vi "Actor Core.vi"(8 "error in":errorcluster, 11 "Interactive Tree in":refnum<class "Interactive Tree.lvclass">) -> (0 "error out":errorcluster, 3 "Actor out":refnum<class "Actor.lvclass">)   [LabVIEW 2016, in "Interactive Tree.lvclass"]
doc: "(<B>Filename</B>: Actor Framework.lvlib:Actor.lvclass:Actor Core.vi)\n\nReceives messages to the actor, reacts to them, and initiates any error handling that may shut the actor down.\n\nDescendant classes may override this VI to append parallel tasks for the actor to complete while it handles messages. Overrides use the Call Parent Method node."
uses:
  Interactive Tree.lvclass
  D:/github/Measure_core/Measure Object/Measure Object.lvclass
  D:/Program Files/National Instruments/LabVIEW 2016/vi.lib/ActorFramework/Actor/Actor.lvclass
  <vilib>/ActorFramework/Actor/Actor.lvclass
  Interactive Tree.lvclass/Interactive Tree.ctl
  Measure Object/Measure Object.lvclass/Measure Object.ctl
  <vilib>/ActorFramework/Actor/Actor.lvclass/Actor.ctl
  <vilib>/ActorFramework/Message Enqueuer/Message Enqueuer.lvclass/Message Enqueuer.ctl
  Interactive Tree Messages/Insert Item Msg/Insert Item Msg.lvclass/Insert Item Msg.ctl
  Measure Object/Read stop event.vi
  <vilib>/ActorFramework/Message Enqueuer/Init from Existing Queue.vi
  <vilib>/ActorFramework/Message Enqueuer/Enqueue.vi
  Interactive Tree Messages/Insert Item Msg/Insert Item Msg.lvclass
  D:/Program Files/National Instruments/LabVIEW 2016/vi.lib/ActorFramework/Message/Message.lvclass
  <vilib>/ActorFramework/Message Priority Queue/Priority Enqueue.vi
  <vilib>/ActorFramework/Message Enqueuer/Message Enqueuer.lvclass
  Measure Object/Measure Object.lvclass
panel:
  in  "Items":i32(listbox)
  in  "Tree":string(tree)
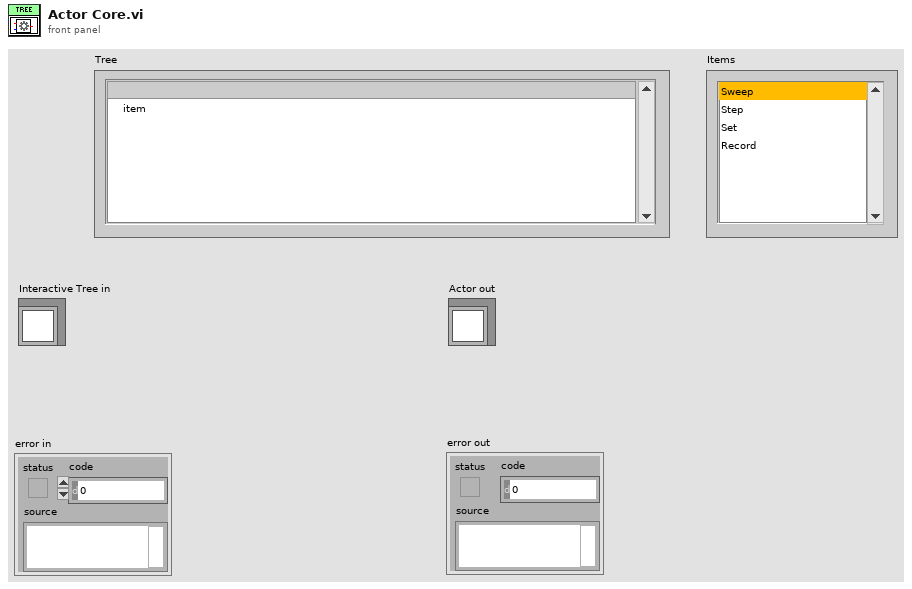
[diagram p1: front panel]
types:
  T1 = typedef "imagedata.ctl" = cluster{"image type":i32, "image depth":i32, "image":u8[], "mask":u8[], "colors":u32[], "Rectangle":cluster{"left":i16, "top":i16, "right":i16, "bottom":i16}}
  T2 = typedef "LVPoint32TypeDef.ctl" = cluster{"Horizontal":i32, "Vertical":i32}
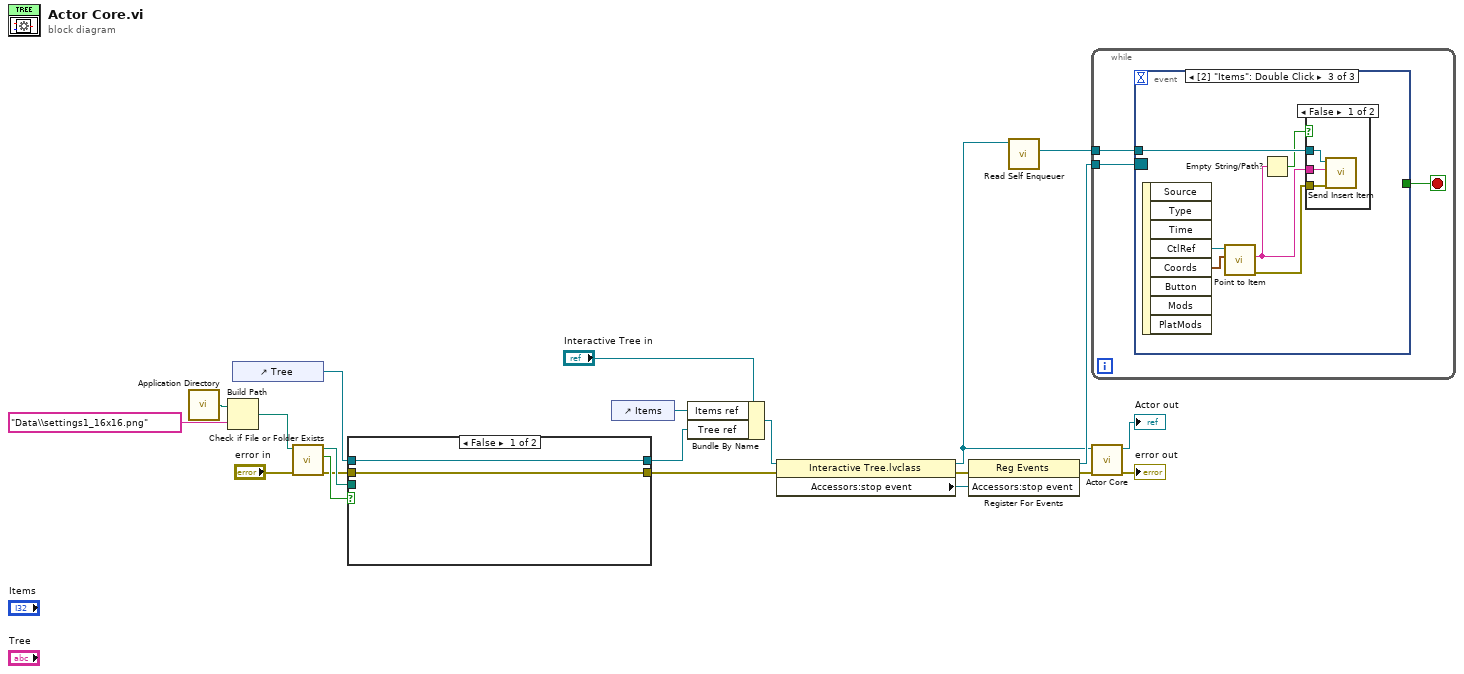
[diagram p0: block diagram]
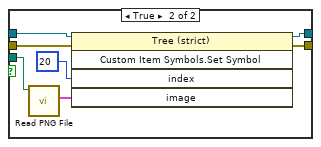
[diagram p2: hidden frame]
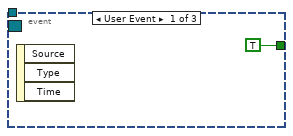
[diagram p3: hidden frame]
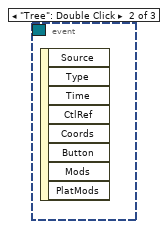
[diagram p4: hidden frame]
diagram:
  n1 = call <vilib>:"Application Directory.vi"() -> ("Application Directory"=w8:path)
  n2 = Build Path(base path=w8, name or relative path="Data\\settings1_16x16.png") -> (appended path=w9:path)
  n3 = control-ref of="Tree"() -> (w5:refnum<vi>)
  n4 = call <vilib>:"Check if File or Folder Exists.vi"("error in (no error)"="error in", "path"=w9) -> ("error out"=w4:errorcluster, "file or folder exists?"=w7:bool, "dup path"=w6:path)  [unwired: 7 in]
  n5 = case shown="False" w7 {
    tunnel: w6 -> [_ w30]
    tunnel: w5 -> [w23 w27]
    tunnel: w4 -> [w22 w26]
    tunnel: [w22 w25] -> w3
    tunnel: [w23 w24] -> w1
    frame False {
    }
    frame True {
      n6 = call <vilib>:"Read PNG File.vi"("path to PNG file"=w30) -> ("image data"=w29:T1)  [unwired: 8 in, 2 out]
      n7 = invoke class="Tree (strict)" method="Custom Item Symbols.Set Symbol"(reference=w27, error in=w26, "index"=20 ("Index"), "image"=w29) -> (reference out=w24:refnum<vi>, error out=w25:errorcluster)  [unwired: 1 in, 3 out]
    }
  }
  n8 = control-ref of="Items"() -> (w11:refnum<vi>)
  n9 = Bundle By Name(cluster="Interactive Tree in", "Items ref"=w11, "Tree ref"=w1) -> (w12:refnum<class "Interactive Tree.lvclass">)
  n10 = property class="Interactive Tree.lvclass"(reference=w12, error in=w3) -> (reference out=w14:refnum<class "Interactive Tree.lvclass">, error out=w16:errorcluster, "Accessors:stop event"=w18:refnum<user-event>)
  n11 = register-events(error in=w16, w18) -> (reference out=w17:refnum<event-registration>, error out=w15:errorcluster)  [unwired: 1 in]
  n12 = call <vilib>:"Read Self Enqueuer.vi"("Actor"=w14) -> ("Self Enqueuer"=w13:refnum<class "Message Enqueuer.lvclass">)  [unwired: 10 in]
  n13 = while {
    tunnel: w17 -> [w33]
    tunnel: w13 -> [w31]
    stop <- w32 stop-if-true
    n14 = event shown="[2] \"Items\": Double Click" {
      selector: w33 -> [_ _ _]
      dyn-events: _ -> [_ _ _]
      timeout: _ -> [_ _ _]
      tunnel: [TRUE _ _] -> w32
      tunnel: w31 -> [_ _ w40]
      event User Event {
        n15 = event-data() -> ()  [unwired: 1 in, 3 out]
      }
      event "Tree": Double Click {
        n16 = event-data() -> ()  [unwired: 1 in, 8 out]
      }
      event "Items": Double Click {
        n17 = event-data() -> ("CtlRef"=w39:refnum<vi>, "Coords"=w38:T2)  [unwired: 1 in, 6 out]
        n18 = call "Point to Item.vi"("Coords"=w38, "reference"=w39) -> ("Error Out"=w37:errorcluster, "Item"=w36:string)  [unwired: 8 in]
        n19 = Empty String/Path?(string/path=w36) -> (empty?=w35:bool)
        n20 = case shown="False" w35 {
          tunnel: w40 -> [w43 _]
          tunnel: w36 -> [w42 _]
          tunnel: w37 -> [w41 _]
          frame False {
            n21 = call "Send Insert Item.vi"("error in (no error)"=w41, "Item"=w42, "Message Enqueuer"=w43) -> ()  [unwired: 7 in, 2 out]
          }
          frame True {
          }
        }
      }
    }
  }
  n22 = call-parent "Actor Core.vi"("error in"=w15, "Measure Object in"=w14) -> ("error out"=→"error out":errorcluster, "Actor out"=→"Actor out":refnum<class "Actor.lvclass">)  [unwired: 8 in]
